vi "写入表头.vi"(8 "错误in":errorcluster caption="错误常量", 11 "各sheet名称数组":string[](array[string])) -> ()   [LabVIEW 2014]
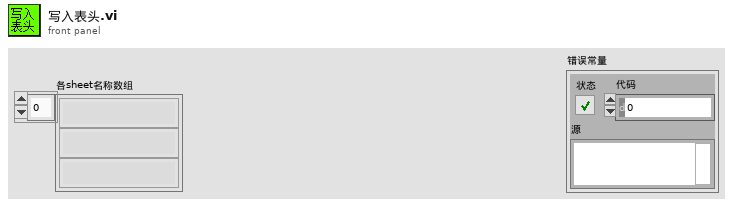
[diagram p1: front panel]
types:
  T1 = typedef "控件-Excel读写选项.ctl" = enum16{"打开表格", "新增sheet", "读取sheet指定位置数据", "读取sheet整个数据", "写入sheet整个数据", "写表头", "数据存到本机", "表格是否开启状态", "关闭表格"}
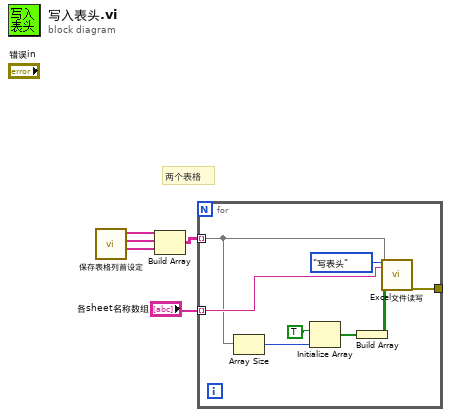
[diagram p0: block diagram]
diagram:
  # "两个表格"
  n1 = call "保存表格列首设定.vi"() -> ("复锁拍螺帽"=w1:string[], "取料拍螺帽"=w2:string[], "拍PCB孔信息"=w5:string[])  [unwired: 9 in]
  n2 = Build Array(w5, w2, w1) -> (w4:string[][])
  n3 = for {
    tunnel: [w13] -> _
    tunnel: "各sheet名称数组" -> [w7] mode=indexing
    tunnel: w4 -> [w6] mode=indexing
    n4 = Array Size(array=w6) -> (size(s)=w11:i32)
    n5 = Initialize Array(TRUE, w11) -> (w10:bool[])
    n6 = Build Array(w10) -> (w9:bool[][])
    n7 = call "Excel文件读写.vi"("选项"=控件-Excel读写选项."写表头", "sheet name"=w7, "列首名称"=w6, "单个结果"=w9) -> ("error out"=w13:errorcluster)  [unwired: 13 in, 2 out]
  }
